vi "STM Write Meta Data (TCP Clst).vi"(6 "Options":T3={"Ignore Timeout Error"=TRUE, "timeout ms (1000)"=1000}, 7 "Meta data":T2[](array[typedef]), 8 "error in":errorcluster, 11 "Connection Info In":T1) -> (0 "error out":errorcluster, 3 "Connection Info Out":T1)   [LabVIEW 2014, in "QwaveSys Raspberry Pi Library.lvlib"]
doc: "Use this VI to transmit the meta data cluster to a remote computer. Sending the meta data to another computer helps maintainability since the data resides only on one side and it is shared to other computers at run time."
uses:
  QwaveSys Raspberry Pi Library.lvlib
  stm_TCP Connection Info.ctl
  _SubVIs/stm_MetaDataElement.ctl
  stm_TCP Write Options.ctl
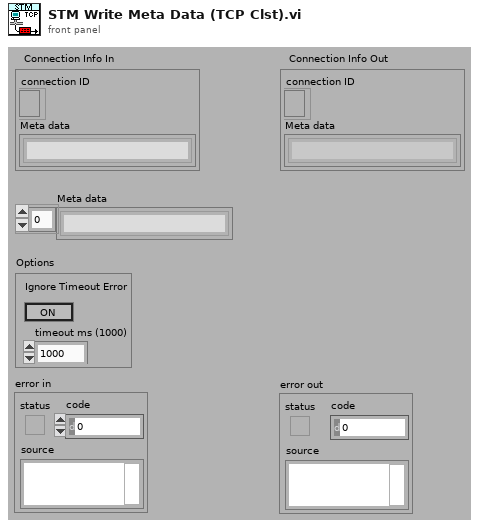
[diagram p1: front panel]
types:
  T1 = typedef "QwaveSys Raspberry Pi Library.lvlib/stm_TCP Connection Info.ctl" = cluster{"connection ID":refnum<k5>, "Meta data":T2[]}
  T2 = typedef "QwaveSys Raspberry Pi Library.lvlib/stm_MetaDataElement.ctl" = string
  T3 = typedef "QwaveSys Raspberry Pi Library.lvlib/stm_TCP Write Options.ctl" = cluster{"Ignore Timeout Error":bool, "timeout ms (1000)":i32}
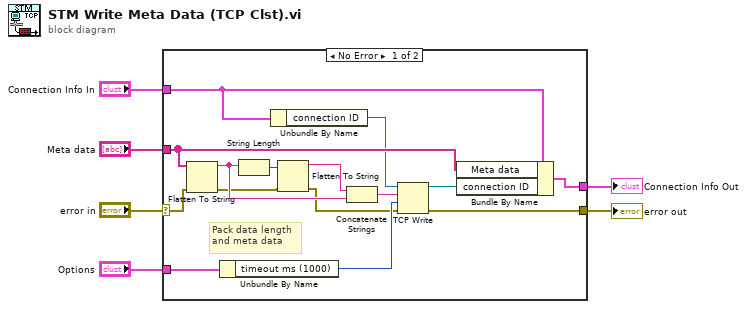
[diagram p0: block diagram]
diagram:
  n1 = case shown="No Error" "error in" {
    selector: "error in" -> [w11 w23]
    tunnel: [w13 w22] -> w6
    tunnel: "Connection Info In" -> [w8 w22]
    tunnel: "Meta data" -> [w12 _]
    tunnel: [w21 w23] -> w4
    tunnel: "Options" -> [w16 _]
    frame No Error {
      # "Pack data length\nand meta data"
      n2 = Flatten To String(anything=w12, error in (no error)=w11) -> (data string=w17:string, error out=w10:errorcluster)  [unwired: 3 out]
      n3 = Unbundle By Name(w16) -> ("timeout ms (1000)"=w15:i32)
      n4 = String Length(string=w17) -> (length=w20:i32)
      n5 = Unbundle By Name(w8) -> ("connection ID"=w7:refnum<k5>)
      n6 = Flatten To String(anything=w20, error in (no error)=w10) -> (data string=w19:string, error out=w9:errorcluster)  [unwired: 3 out]
      n7 = Concatenate Strings(w19, w17) -> (w18:string)
      n8 = TCP Write(connection ID=w7, data in=w18, error in (no error)=w9, 9:w15) -> (connection ID out=w14:refnum<k5>, error out=w21:errorcluster)  [unwired: 1 out]
      n9 = Bundle By Name(cluster=w8, "Meta data"=w12, "connection ID"=w14) -> (w13:T1)
    }
    frame Error {
    }
  }
  "Connection Info Out" <- w6
  "error out" <- w4
